vi "Quick Load Audio File.vi"(8 "error in (no error)":errorcluster, 10 "Codec":string, 11 "Path":path) -> (0 "error out":errorcluster, 1 "data":waveform(i16)[](array[waveform]), 2 "Sample Rate (Hz)":u32, 3 "Channels":u32, 5 "Length (Samples)":u64)   [LabVIEW 2020, in "G-Audio.lvlib"]
doc: "A single VI method to load an entire audio file from disk. The audio data will be returned as an I16 waveform array.\n\nNote this method is faster than reading audio chunks in a loop, but can result in higher peak memory allocation. If the file is very large, LabVIEW may run out of memory. If <b>codec</b> isn't specified, file extension determines the codec type.\n\nSupported codecs: flac, mp3, ogg (vorbis), and wav."
uses:
  G-Audio.lvlib
  Private/Get File Extension (Reentrant).vi
  <vilib>/Utility/error.llb/Error Cluster From Error Code.vi
  lib/g_audio_x86.dll
  lib/g_audio_x64.dll
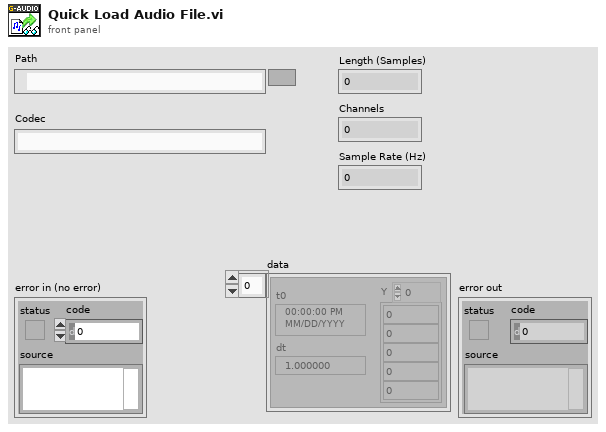
[diagram p1: front panel]
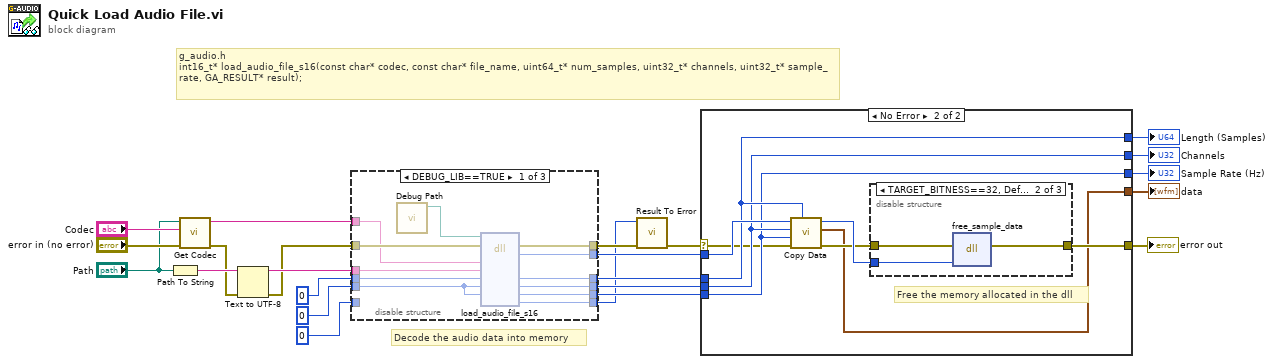
[diagram p0: block diagram]
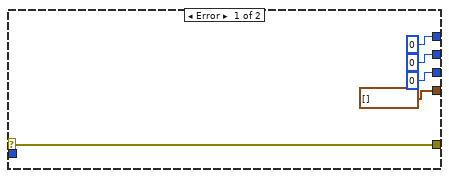
[diagram p2: hidden frame]
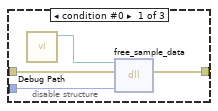
[diagram p3: hidden frame]
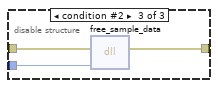
[diagram p4: hidden frame]
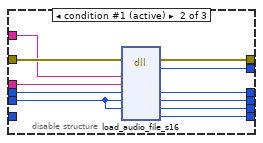
[diagram p5: hidden frame]
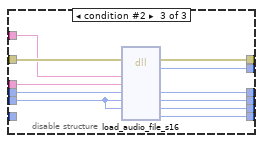
[diagram p6: hidden frame]
diagram:
  # "g_audio.h\nint16_t* load_audio_file_s16(const char* codec, const char* file_name, uint64_t* num_samples, uint32_t* channels, uint32_t* sample_rate, GA_RESULT* result);"
  # "Decode the audio data into memory"
  n1 = Path To String(path="Path") -> (string=w5:string)
  n2 = call "Get Codec.vi"("error in (no error)"="error in (no error)", "Codec In"="Codec", "Absolute Path"="Path") -> ("error out"=w3:errorcluster, "Codec Out"=w10:string)  [unwired: 7 in]
  n3 = Text to UTF-8(8:w3, 11:w5) -> (0:w2:errorcluster, 3:w4:string)  [unwired: 1 in]
  n4 = disable-structure shown="DEBUG_LIB==TRUE" {
    disable-tunnel: w2 -> [w35 w46 w57]
    disable-tunnel: [w33 w44 w55] -> w20
    disable-tunnel: [w32 w43 w54] -> w19
    disable-tunnel: [w31 w42 w53] -> w18
    disable-tunnel: w4 -> [w29 w40 w51]
    disable-tunnel: [w25 w36 w47] -> w17
    disable-tunnel: [w34 w45 w56] -> w8
    disable-tunnel: u32 0 ("num_samples") -> [w30 w41 w52]
    disable-tunnel: u64 0 ("num_samples") -> [w28 w39 w50]
    disable-tunnel: 0 ("num_samples") -> [_ _ _]
    disable-tunnel: [w26 w37 w48] -> w7
    disable-tunnel: w10 -> [w27 w38 w49]
    frame condition #0 {
      n5 = call "Debug Path.vi"() -> ("Debug Path"=w24:path)  [unwired: 11 in]
      n6 = dll-call lib="?" fn="load_audio_file_s16"(path in=w24, error in=w35, "codec"=w27, "file_name"=w29, "num_samples"=w28, "channels"=w30, "sample_rate"=w30) -> (error out=w34:errorcluster, "sample_data"=w25:i64, "num_samples"=w33:u64, "channels"=w32:u32, "sample_rate"=w31:u32, "result"=w26:i32)  [unwired: 4 in, 1 out]
    }
    frame condition #1 (active) {
      n7 = dll-call lib="C:/github/dataflowg/g-audio/src/LabVIEW/G-Audio/lib/g_audio_x86.*" fn="load_audio_file_s16"(error in=w46, "codec"=w38, "file_name"=w40, "num_samples"=w39, "channels"=w41, "sample_rate"=w41) -> (error out=w45:errorcluster, "sample_data"=w36:i64, "num_samples"=w44:u64, "channels"=w43:u32, "sample_rate"=w42:u32, "result"=w37:i32)  [unwired: 5 in, 1 out]
    }
    frame condition #2 {
      n8 = dll-call lib="C:/github/dataflowg/g-audio/src/LabVIEW/G-Audio/lib/g_audio_x64.*" fn="load_audio_file_s16"(error in=w57, "codec"=w49, "file_name"=w51, "num_samples"=w50, "channels"=w52, "sample_rate"=w52) -> (error out=w56:errorcluster, "sample_data"=w47:i64, "num_samples"=w55:u64, "channels"=w54:u32, "sample_rate"=w53:u32, "result"=w48:i32)  [unwired: 5 in, 1 out]
    }
  }
  n9 = call "Result To Error.vi"("error in (no error)"=w8, "Result Code"=w7) -> ("error out"=w6:errorcluster)  [unwired: 9 in]
  n10 = case shown="No Error" w6 {
    selector: w6 -> [w58 w63]
    tunnel: [w58 w71] -> w23
    tunnel: w20 -> [_ w67]
    tunnel: w19 -> [_ w66]
    tunnel: w18 -> [_ w65]
    tunnel: w17 -> [_ w70]
    tunnel: [waveform(i16)[] [] ("Waveform Data") w64] -> w16
    tunnel: [u64 0 ("num_samples") w67] -> w14
    tunnel: [u32 0 ("channels") w66] -> w13
    tunnel: [u32 0 ("sample_rate") w65] -> w12
    frame Error {
    }
    frame No Error {
      # "Free the memory allocated in the dll"
      n11 = call "Copy Data.vi"("num_samples"=w67, "error in (no error)"=w63, "sample_rate"=w65, "channels"=w66, "Data Pointer in"=w70) -> ("error out"=w68:errorcluster, "Waveform Data"=w64:waveform(i16)[], "Data Pointer out"=w69:i64)  [unwired: 4 in]
      n12 = disable-structure shown="TARGET_BITNESS==32, Default" {
        disable-tunnel: [w75 w78 w81] -> w71
        disable-tunnel: w69 -> [w74 w77 w80]
        disable-tunnel: w68 -> [w73 w76 w79]
        frame condition #0 {
          n13 = call "Debug Path.vi"() -> ("Debug Path"=w72:path)  [unwired: 11 in]
          n14 = dll-call lib="?" fn="free_sample_data"(path in=w72, error in=w73, "Address (Pointer)"=w74) -> (error out=w75:errorcluster)  [unwired: 3 in, 1 out]
        }
        frame condition #1 (active) {
          n15 = dll-call lib="C:/github/dataflowg/g-audio/src/LabVIEW/G-Audio/lib/g_audio_x86.*" fn="free_sample_data"(error in=w76, "Address (Pointer)"=w77) -> (error out=w78:errorcluster)  [unwired: 4 in, 1 out]
        }
        frame condition #2 {
          n16 = dll-call lib="C:/github/dataflowg/g-audio/src/LabVIEW/G-Audio/lib/g_audio_x64.*" fn="free_sample_data"(error in=w79, "Address (Pointer)"=w80) -> (error out=w81:errorcluster)  [unwired: 4 in, 1 out]
        }
      }
    }
  }
  "error out" <- w23
  "Length (Samples)" <- w14
  "Channels" <- w13
  "Sample Rate (Hz)" <- w12
  "data" <- w16
